vi "ConfigureHTTP(subVI).vi"(8 "error in (no error)":errorcluster) -> (0 "error out":errorcluster, 3 "Refnum out":T1)   [LabVIEW 2017]
uses:
  <vilib>/httpClient/ClientHandle.ctl
  <vilib>/httpClient/POSTBuffer.vi
  <vilib>/httpClient/LabVIEWHTTPClient.lvlib
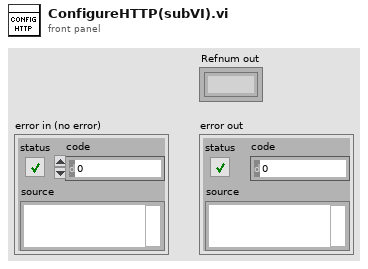
[diagram p1: front panel]
types:
  T1 = typedef "LabVIEWHTTPClient.lvlib/ClientHandle.ctl" = refnum<k1>
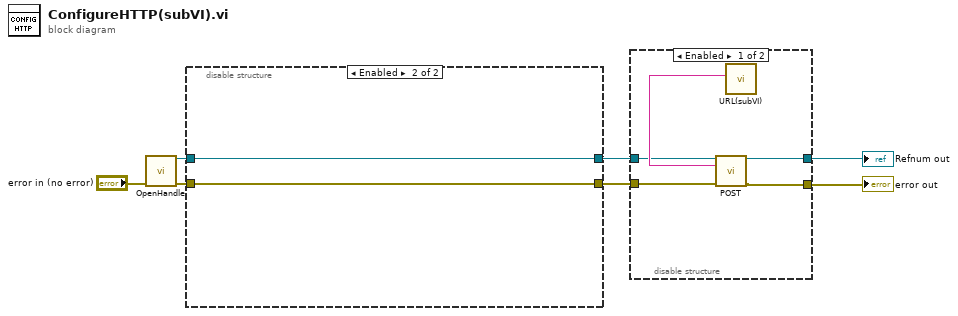
[diagram p0: block diagram]
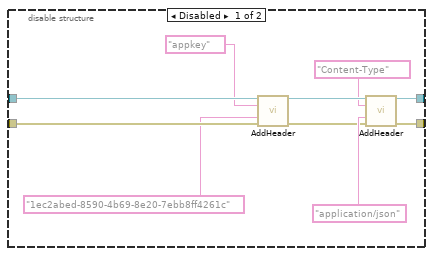
[diagram p3: hidden frame]
diagram:
  n1 = call <vilib>:"OpenHandle.vi"("error in (no error)"="error in (no error)") -> ("client handle out"=w6:T1, "error out"=w5:errorcluster)  [unwired: 13 in]
  n2 = disable-structure shown="Enabled" {
    disable-tunnel: w6 -> [w17 w19]
    disable-tunnel: w5 -> [w16 w18]
    disable-tunnel: [w15 w19] -> w4
    disable-tunnel: [w14 w18] -> w3
    frame Disabled {
      n3 = call <vilib>:"AddHeader.vi"("client handle"=w17, "header"="appkey", "value"="1ec2abed-8590-4b69-8e20-7ebb8ff4261c", "error in (no error)"=w16) -> ("client handle out"=w13:T1, "error out"=w10:errorcluster)  [unwired: 10 in]
      n4 = call <vilib>:"AddHeader.vi"("client handle"=w13, "header"="Content-Type", "value"="application/json", "error in (no error)"=w10) -> ("client handle out"=w15:T1, "error out"=w14:errorcluster)  [unwired: 10 in]
    }
    frame Enabled {
    }
  }
  n5 = disable-structure shown="Enabled" {
    disable-tunnel: w4 -> [w23 w26]
    disable-tunnel: w3 -> [w22 w25]
    disable-tunnel: [w21 w25] -> w2
    disable-tunnel: [w20 w26] -> w1
    frame Enabled {
      n6 = call "URL(subVI).vi"() -> ("URL"=w24:string)  [unwired: 11 in]
      n7 = call-poly <vilib>:"POST.vi"("client handle"=w23, "url"=w24, "error in (no error)"=w22) -> ("client handle out"=w20:T1, "error out"=w21:errorcluster)  [unwired: 9 in, 2 out]
    }
    frame Disabled {
    }
  }
  "error out" <- w2
  "Refnum out" <- w1
